vi "Main.vi"(8 "error in (no error)":errorcluster) -> (0 "error out":errorcluster)   [LabVIEW 2014, in "Display Module.lvlib"]
uses:
  Display Module.lvlib
  Queue FGV.ctl
  Message.ctl
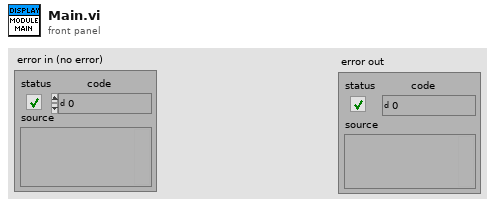
[diagram p1: front panel]
types:
  T1 = typedef "Display Module.lvlib/Queue FGV.ctl" = enum16{"Set", "Get", "Release"}
  T2 = typedef "Display Module.lvlib/Message.ctl" = cluster{"Message":enum16{"Initialise", "Error", "Close"}, "Data":variant}
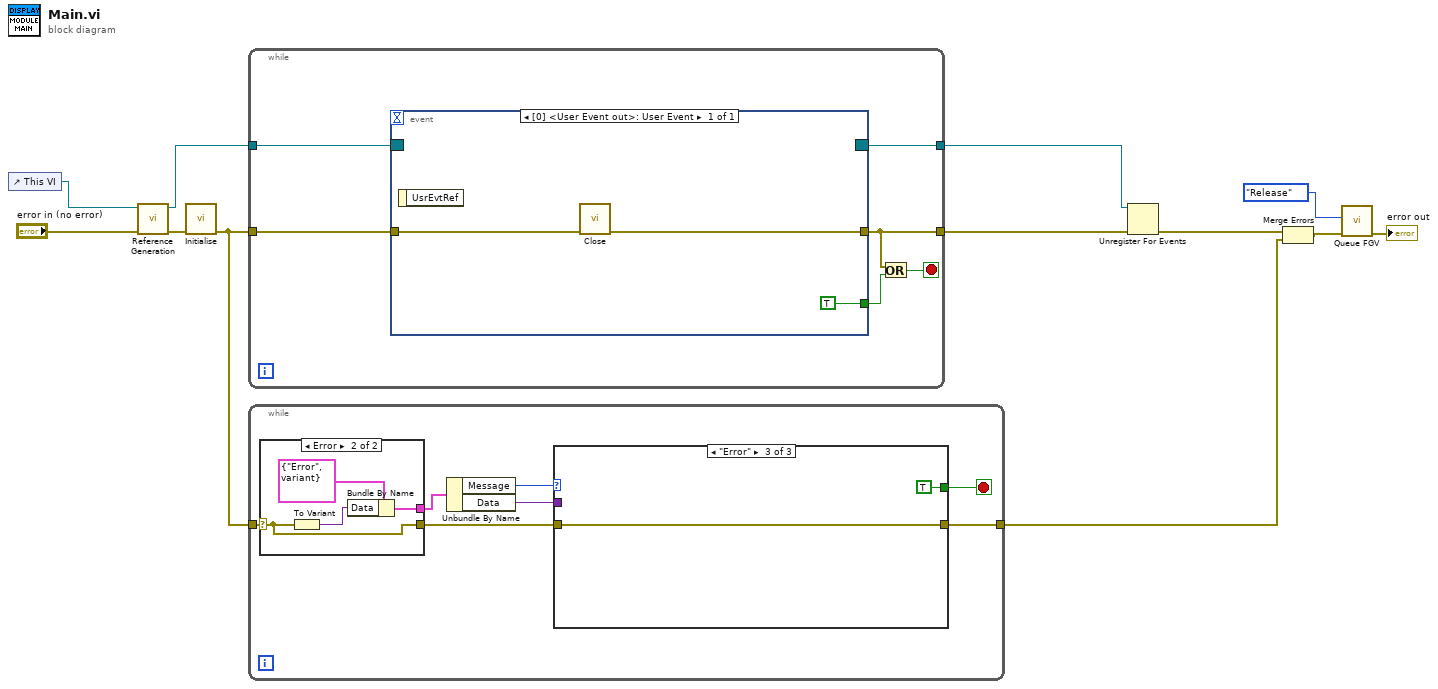
[diagram p0: block diagram]
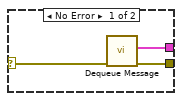
[diagram p2: hidden frame]
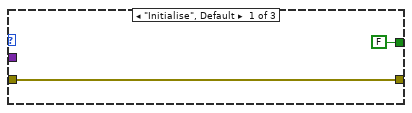
[diagram p3: hidden frame]
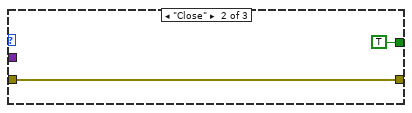
[diagram p4: hidden frame]
diagram:
  n1 = control-ref of="This VI"() -> (w12:refnum<vi>)
  n2 = call "Reference Generation.vi"("error in (no error)"="error in (no error)", "VI in"=w12) -> ("error out"=w10:errorcluster, "User Events Reference"=w9:refnum<event-registration>)  [unwired: 8 in]
  n3 = call "Initialise.vi"("error in (no error)"=w10) -> ("error out"=w8:errorcluster)  [unwired: 10 in]
  n4 = while {
    tunnel: w9 -> [w18]
    tunnel: w8 -> [w17]
    tunnel: [w16] -> w7
    tunnel: [w15] -> w6
    stop <- w13 stop-if-true
    n5 = event shown="[0] <User Event out>: User Event" {
      selector: w18 -> [_]
      dyn-events: [_] -> w16
      timeout: _ -> [_]
      tunnel: w17 -> [w21]
      tunnel: [TRUE] -> w14
      tunnel: [w19] -> w15
      event User Event {
        n6 = event-data() -> ()  [unwired: 1 in, 1 out]
        n7 = call "Close.vi"("error in (no error)"=w21) -> ("error out"=w19:errorcluster)  [unwired: 10 in]
      }
    }
    n8 = Or(x=w15, y=w14) -> (x .or. y?=w13:bool)
  }
  n9 = while {
    tunnel: w8 -> [w27]
    tunnel: [w22] -> w3
    stop <- w24 stop-if-true
    n10 = case shown="Error" w27 {
      selector: w27 -> [w31 w33]
      tunnel: [w30 w33] -> w25
      tunnel: [w29 w32] -> w23
      frame No Error {
        n11 = call "Dequeue Message.vi"("error in (no error)"=w31) -> ("error out"=w30:errorcluster, "output cluster"=w29:T2)  [unwired: 8 in, 1 out]
      }
      frame Error {
        n12 = To Variant(anything=w33) -> (Variant=w34:variant)
        n13 = Bundle By Name(cluster=T2 {"Message"=enum."Error", "Data"=variant} ("output cluster"), "Data"=w34) -> (w32:T2)
      }
    }
    n14 = Unbundle By Name(w23) -> ("Message"=w28:enum16{"Initialise", "Error", "Close"}, "Data"=w26:variant)
    n15 = case shown="\"Error\"" w28 {
      tunnel: w26 -> [_ _ _]
      tunnel: w25 -> [w37 w39 w40]
      tunnel: [w37 w39 w40] -> w22
      tunnel: [FALSE ("event data") TRUE ("event data") TRUE ("event data")] -> w24
      frame "Initialise", Default {
      }
      frame "Close" {
      }
      frame "Error" {
      }
    }
  }
  n16 = Unregister For Events(event registration refnum=w7, error in=w6) -> (error out=w5:errorcluster)
  n17 = Merge Errors(w5, w3) -> (w4:errorcluster)
  n18 = call "Queue FGV.vi"("error in (no error)"=w4, "Action"=Queue_FGV."Release") -> ("error out"=→"error out":errorcluster)  [unwired: 8 in, 1 out]
